vi "rmx13_rx.vi"() -> ()   [LabVIEW 2011]
panel:
  in  "stop":bool
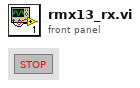
[diagram p1: front panel]
types:
  T1 = cluster{"up":bool, "down":bool, "left":bool, "right":bool, "xup":bool, "xdown":bool, "hup":bool, "hdown":bool, "xfwd":bool, "xback":bool, "forward angular velocity":dbl, "forward angular velocity":dbl, "Knob":dbl}
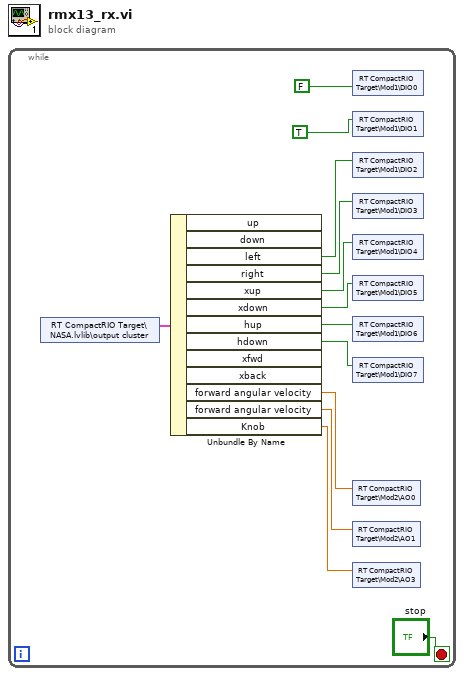
[diagram p0: block diagram]
diagram:
  n1 = while {
    stop <- "stop" stop-if-true
    n2 = shared-variable "RT CompactRIO Target\\NASA.lvlib\\output cluster"() -> (w12:T1)  [unwired: 1 in, 1 out]
    n3 = Unbundle By Name(w12) -> ("left"=w8:bool, "right"=w7:bool, "xup"=w6:bool, "xdown"=w5:bool, "hup"=w4:bool, "hdown"=w3:bool, "forward angular velocity"=w11:dbl, "forward angular velocity"=w10:dbl, "Knob"=w9:dbl)  [unwired: 4 out]
    n4 = shared-variable "RT CompactRIO Target\\Mod1\\DIO0"(FALSE) -> ()  [unwired: 1 in, 1 out]
    n5 = shared-variable "RT CompactRIO Target\\Mod1\\DIO1"(TRUE) -> ()  [unwired: 1 in, 1 out]
    n6 = shared-variable "RT CompactRIO Target\\Mod1\\DIO2"(w8) -> ()  [unwired: 1 in, 1 out]
    n7 = shared-variable "RT CompactRIO Target\\Mod1\\DIO3"(w7) -> ()  [unwired: 1 in, 1 out]
    n8 = shared-variable "RT CompactRIO Target\\Mod1\\DIO4"(w6) -> ()  [unwired: 1 in, 1 out]
    n9 = shared-variable "RT CompactRIO Target\\Mod1\\DIO5"(w5) -> ()  [unwired: 1 in, 1 out]
    n10 = shared-variable "RT CompactRIO Target\\Mod1\\DIO6"(w4) -> ()  [unwired: 1 in, 1 out]
    n11 = shared-variable "RT CompactRIO Target\\Mod1\\DIO7"(w3) -> ()  [unwired: 1 in, 1 out]
    n12 = shared-variable "RT CompactRIO Target\\Mod2\\AO0"(w11) -> ()  [unwired: 1 in, 1 out]
    n13 = shared-variable "RT CompactRIO Target\\Mod2\\AO1"(w10) -> ()  [unwired: 1 in, 1 out]
    n14 = shared-variable "RT CompactRIO Target\\Mod2\\AO3"(w9) -> ()  [unwired: 1 in, 1 out]
  }
